vi "BPZ V1.5.vi"() -> ()   [LabVIEW 2025]
uses:
  StatesV2.0.ctl
  runningPhaseV2.0.ctl
  CommandsV2.0.ctl
  <vilib>/Analysis/3filter.llb/Filter Passband Type.ctl
  <vilib>/Utility/error.llb/DialogType.ctl
  <vilib>/Utility/file.llb/Write Delimited Spreadsheet (DBL).vi
  <vilib>/Instr/_visa.llb/VISA Configure Serial Port (Instr).vi
  <vilib>/Analysis/NI_AALBase.lvlib
  <vilib>/ptbypt/NI_PtbyPt.lvlib
panel:
  out "Time working":dbl format="%<%H:%M:%S>t"
  out "State":T1
  out "Current time":timestamp format="%<%H:%M:%S\n%x>T"
  in  "Em. Stop":bool
  out "Drive torque [mNm]":dbl(knob)=4657.939556380271 scale=0.0..1000.0 scale format="%#_2f"
  out "Motor velocity [RPM]":dbl(knob) scale=0.0..800.0
  out "Motor current [A]":dbl(knob) scale=0.0..5.0
  out "Gear temperature":dbl(slide)=24.329999999999984 scale=0.0..200.0
  out "Amb. temperature":dbl(slide)=24.970000000000027 scale=0.0..50.0
  out "Noise level [dB]":dbl(knob)=36.22 scale=0.0..120.0
  out "Automatic on":bool
  out "UART status":bool=TRUE
  out "Pump 1 engaged":bool
  out "Pump 2 engaged":bool
  out "Logging":bool
  out "Drive on":bool
  out "EPOS Status":bool=TRUE
  in  "?":T2(tab)=enum."Settings"
  in  "Connect":bool
  in  "Disconnect":bool
  in  "Connect":bool
  in  "Disconnect":bool
  in  "Pump 1":bool
  in  "Pump 2":bool
  in  "Filename":string
  in  "Ready":bool
  in  "Log folder":path
  in  "AutoStop":bool
  in  "AutoStart":bool
  in  "Enable logging":bool
  in  "Current filter":bool
  in  "Array":cluster{"RPM":u16, "TIME [s]":u32}[](array[cluster])
  out "targetRPM":i32
  out "cyclesCompleted":i32
  out "cyclesToComplete":i32
  out "runningPhase":T3
  out "ETA":u32 format="%<%H:%M:%S>t"
  in  "Communication settings":T4={"Device"="EPOS4", "Protocol stack "="MAXON SERIAL V2", "Interface"="USB", "Port"="USB0", "Baud rate"=1000000, "Timeout [ms]"=500}
  in  "Velocity profile":T5={"Acceleration [rpm/s]"=1060, "Deceleration  [rpm/s]"=1060}
  in  "UART Settings":T6={"Flow control"=0, "Stop bits"=10, "Parity bit"=enum."None", "Data bits"=8, "Baud rate"=115200, "Port"="COM3"} {"Stop bits" items=["1.0"=10, "1.5"=15, "2.0"=20]; "Flow control" items=["None", "XON/XOFF", "RTS/CTS", "XON/XOFF & RTS/CTS", "DTR/DSR", "XON/XOFF & DTR/DSR"]}
  in  "Surface emmisivity":dbl=1.0 min=0.05 max=1.0 step=0.05 format="%#.2g"
  in  "Torque constant [mNm/mA]":dbl=0.0273
  in  "Motor gear ratio":dbl=5.3076
  in  "Belt drive ratio":dbl=1.5
  in  "Motor gear efficiency":dbl=0.9
  in  "Belt drive efficiency":dbl=0.95 min=0.89 max=0.99 step=0.01
  in  "Speed setting [RPM]":dbl=60.0 min=0.0 max=750.0 step=10.0
  in  "Stop motor":bool
  in  "Start motor":bool
  in  "Stop logging":bool
  in  "Start logging":bool
  in  "?":T7(tab)
  out "Velocity [RPM]":cluster{dbl[], dbl[]}(graph)
  out "Torque [mNm]":cluster{dbl[], dbl[]}(graph)
  out "Noise [dB]":cluster{dbl[], dbl[]}(graph)
  out "Temperature [degC]":cluster{dbl[], dbl[]}[](graph)
  in  "QUIT":bool
  # "Current status"
  # "EPOS connection control"
  # "UART connection control"
  # "Pump control"
  # "Options"
  # "Start/Stop"
  # "EPOS Settings"
  # "UART Settings"
  # "Motor control"
  # "Logger control"
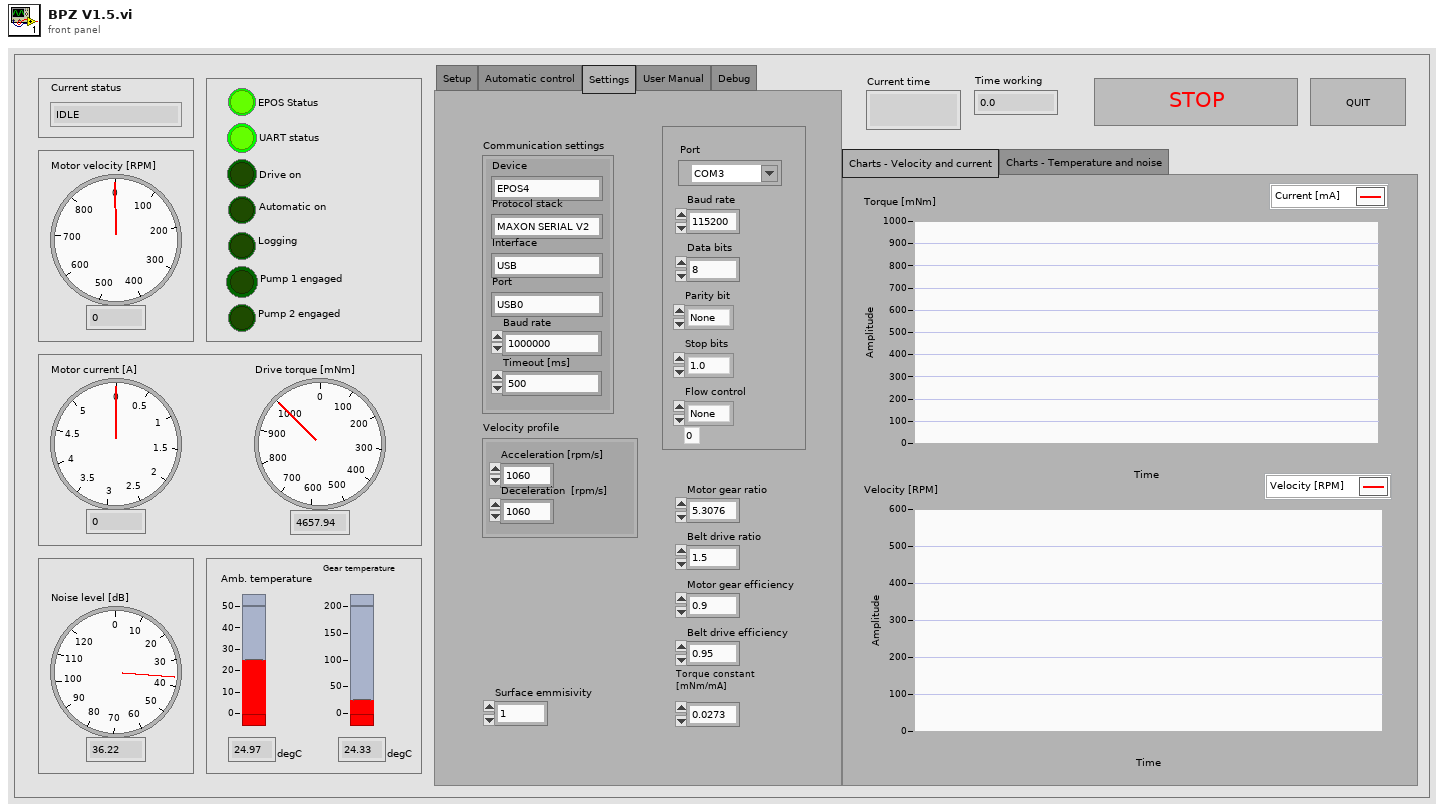
[diagram p1: front panel]
types:
  T1 = typedef "StatesV2.0.ctl" = enum16{"IDLE", "READY", "RUNNING", "ERROR", "SHUTDOWN"}
  T2 = enum32{"Setup", "Automatic control", "Settings", "User Manual", "Debug"}
  T3 = typedef "runningPhaseV2.0.ctl" = enum16{"DISABLED", "INITIALIZE_CYCLE", "START_MOTOR", "COUNTDOWN", "STOP_MOTOR", "CYCLE_COMPLETE"}
  T4 = cluster{"Device":string, "Protocol stack ":string, "Interface":string, "Port":string, "Baud rate":u32, "Timeout [ms]":u32}
  T5 = cluster{"Acceleration [rpm/s]":u32, "Deceleration  [rpm/s]":u32}
  T6 = cluster{"Flow control":u16, "Stop bits":u16, "Parity bit":enum16{"None", "Odd", "Even", "Mark", "Space"}, "Data bits":u16, "Baud rate":u32, "Port":refnum<visa-resource-name>}
  T7 = enum32{"Charts - Velocity and current", "Charts - Temperature and noise"}
  T8 = cluster{"UART":cluster{"Amb. temp":dbl[], "Gear temp":dbl[], "Noise lvl":dbl[], "time":dbl[]}, "EPOS":cluster{"Speed":dbl[], "Torque":dbl[], "time":dbl[]}}
  T9 = typedef "CommandsV2.0.ctl" = enum16{"No_Command", "Ready", "Initialize_Cycle", "Stop", "SHUTDOWN", "EPOS_Connect", "EPOS_Disconnect", "UART_Connect", "UART_Disconnect", "Pump1_Toggle", "Pump2_Toggle"}
  T10 = cluster{"Speed":dbl[], "Torque":dbl[], "time":dbl[]}
  T11 = typedef "NI_AALBase.lvlib/Filter Passband Type.ctl" = enum32{"Lowpass", "Highpass", "Bandpass", "Bandstop"}
  T12 = cluster{"Gear temp":dbl, "Amb temp":dbl, "Noise lvl":dbl, "Torque":dbl, "RPM":dbl, "Time":dbl}
  T13 = cluster{"isLoggingEnabled":bool, "isUARTConnected":bool, "isEPOSConnected ":bool, "lastCommand":T9, "cyclesToComplete":i32, "targetRPM":i32, "axisHandle":cluster{"keyHandle":u32, "nodeId":u16}, "VISA resource name":refnum<visa-resource-name>, "isMotorOn":bool, "runningPhase":T3, "cyclesCompleted":i32, "isPump1on":bool, "isPump2on":bool, "timeToComplete":u32, "lastNotifyMs":u32, "UARTStartTime":timestamp, "MotorStartTime":timestamp, "ETA":u32}
  T14 = cluster{"Amb. temp":dbl[], "Gear temp":dbl[], "Noise lvl":dbl[], "time":dbl[]}
  T15 = cluster{"array type (2D Dbl)[0]":dbl, "array type (2D Dbl)[1]":dbl, "array type (2D Dbl)[2]":dbl}
  T16 = typedef "DialogType.ctl" = u16
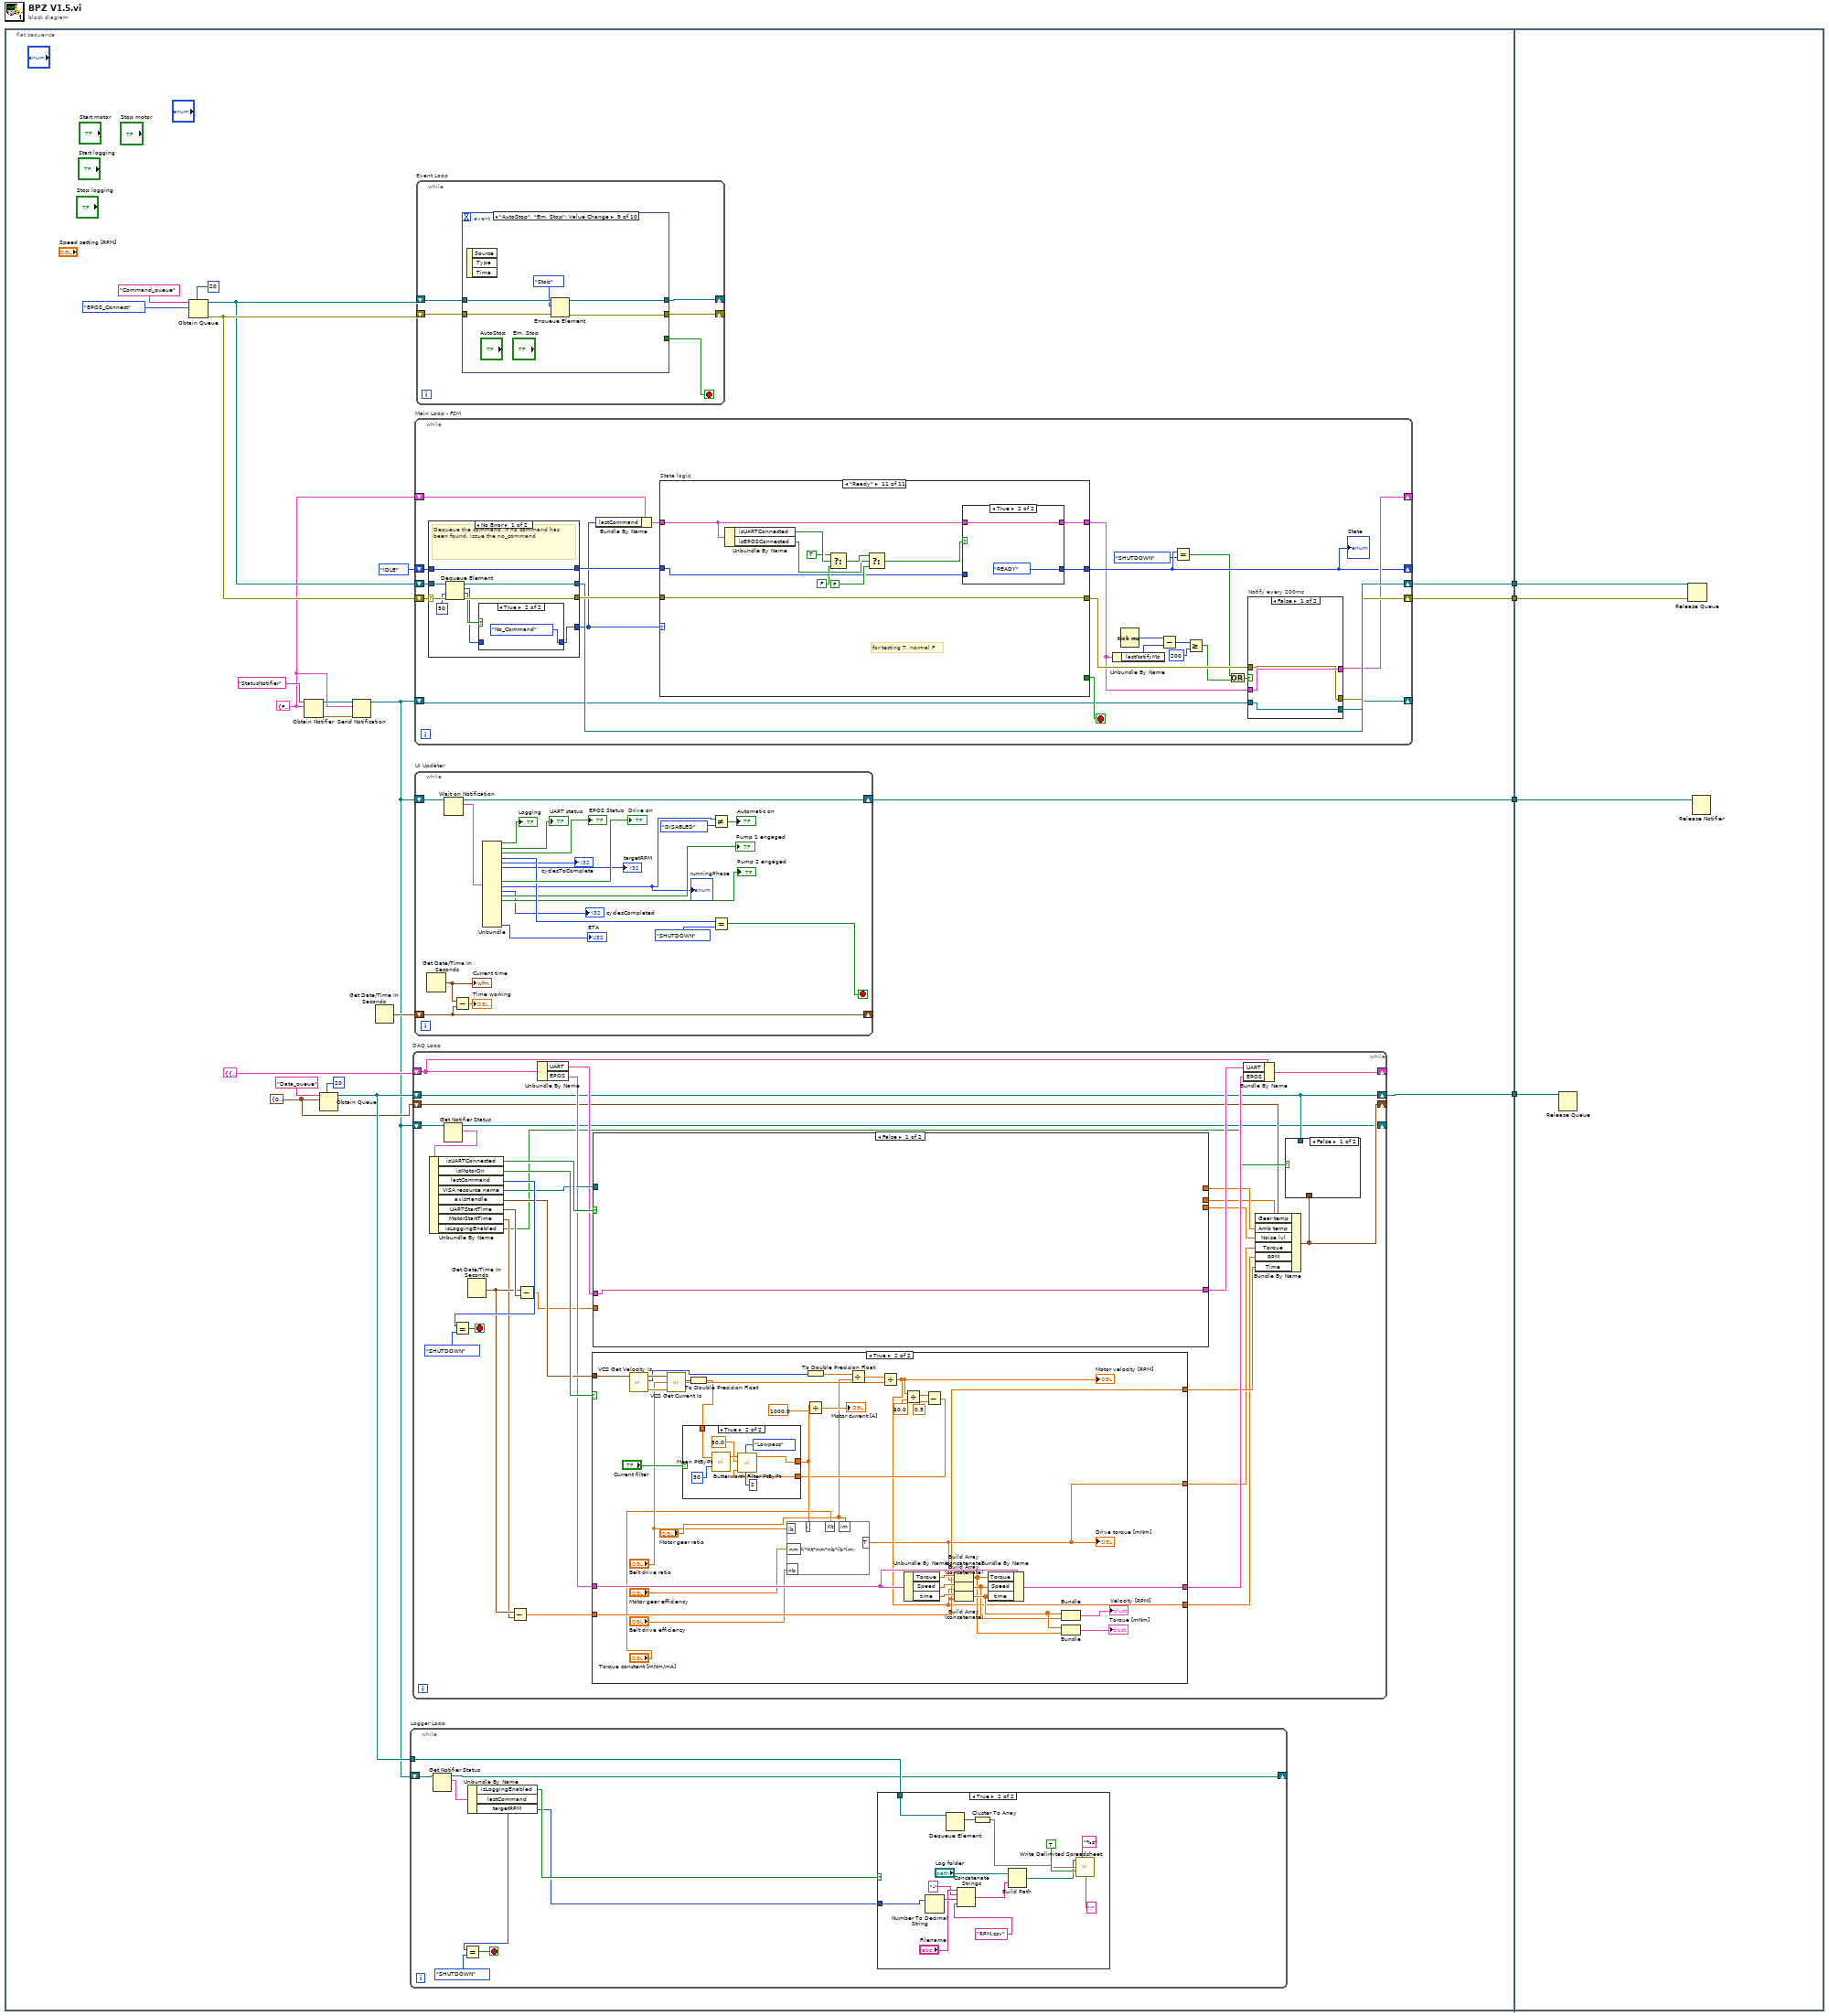
[diagram p0: block diagram]
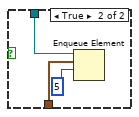
[diagram p3: hidden frame]
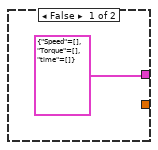
[diagram p4: hidden frame]
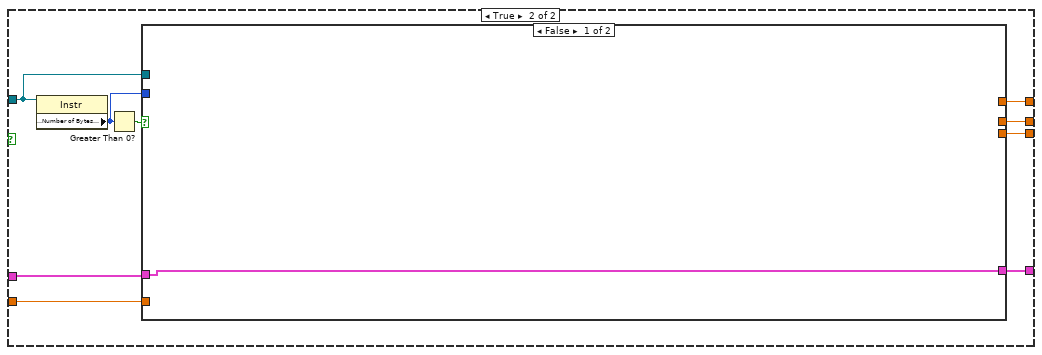
[diagram p6: hidden frame]
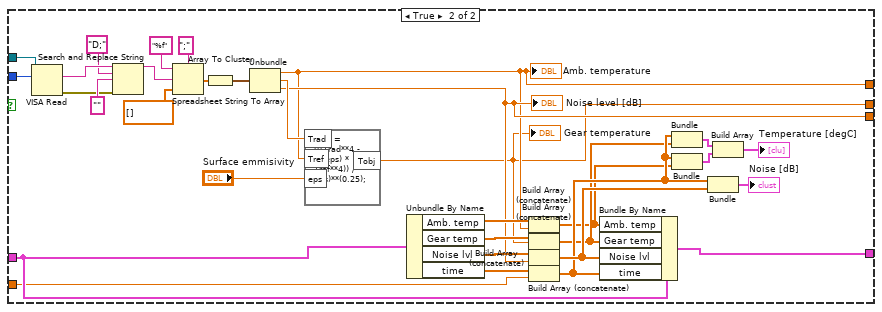
[diagram p7: hidden frame]
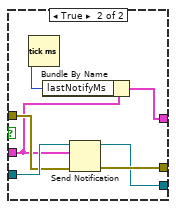
[diagram p8: hidden frame]
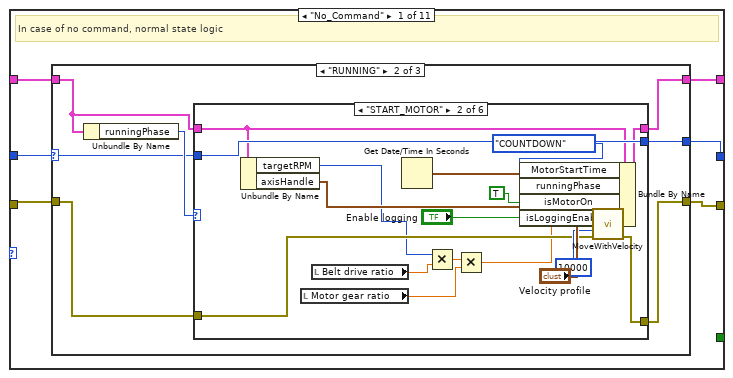
[diagram p9: hidden frame]
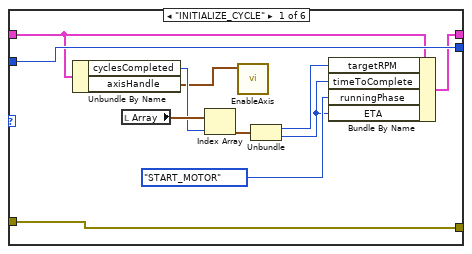
[diagram p11: hidden frame]
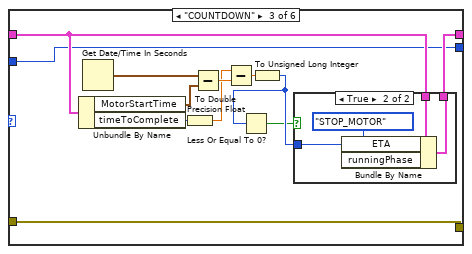
[diagram p12: hidden frame]
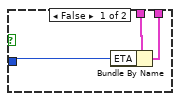
[diagram p13: hidden frame]
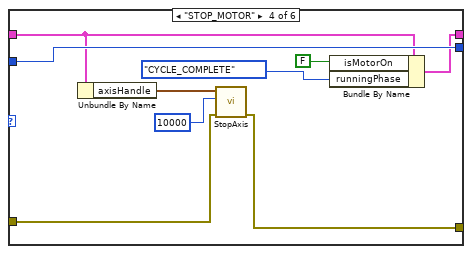
[diagram p14: hidden frame]
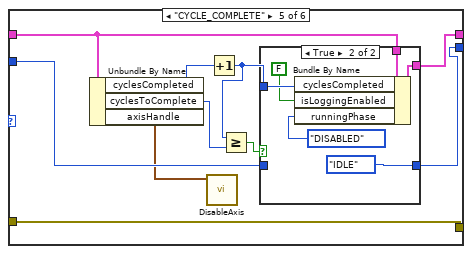
[diagram p15: hidden frame]
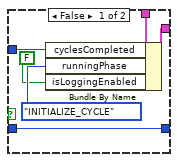
[diagram p16: hidden frame]
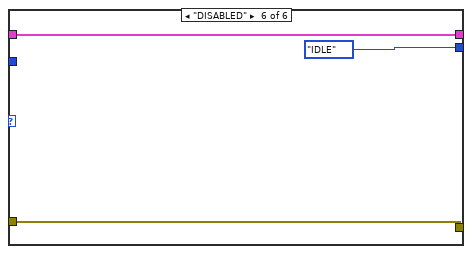
[diagram p17: hidden frame]
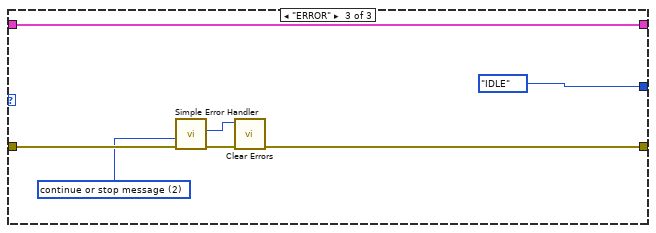
[diagram p18: hidden frame]
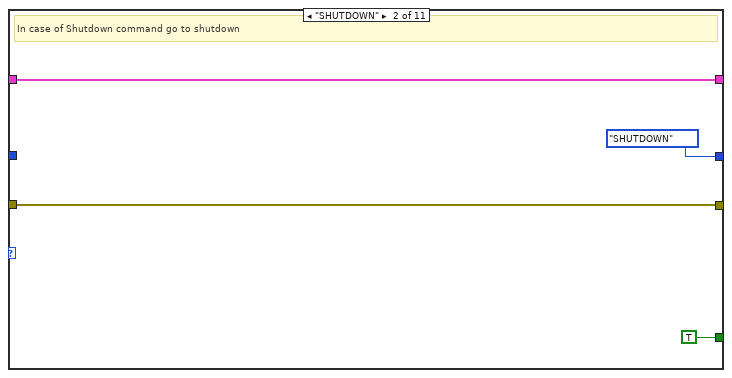
[diagram p19: hidden frame]
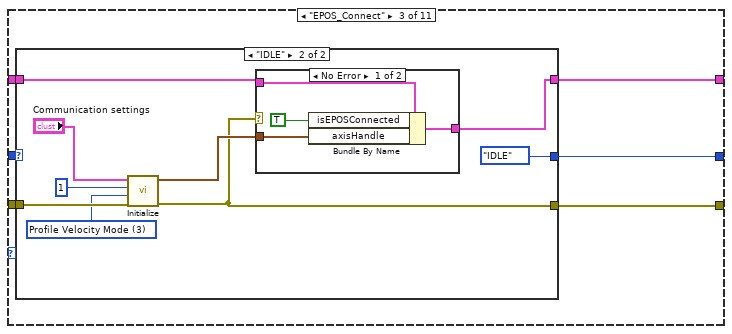
[diagram p20: hidden frame]
diagram:
  n1 = flat-sequence {
    tunnel: [w19] -> w4
    tunnel: [w7] -> w3
    tunnel: [w6] -> w2
    tunnel: [w5] -> w1
    tunnel: w4 -> [w550]
    tunnel: w3 -> [w549]
    tunnel: w2 -> [w548]
    tunnel: w1 -> [w547]
    frame #0 {
      w14 = T12 {"Gear temp"=0.0, "Amb temp"=0.0, "Noise lvl"=0.0, "Torque"=0.0, "RPM"=0.0, "Time"=0.0}
      w8 = T13 {"isLoggingEnabled"=FALSE, "isUARTConnected"=FALSE, "isEPOSConnected "=FALSE, "lastCommand"=enum."No_Command", "cyclesToComplete"=0, "targetRPM"=0, "axisHandle"={"keyHandle"=0, "nodeId"=1}, "VISA resource name"="", "isMotorOn"=FALSE, "runningPhase"=enum."DISABLED", "cyclesCompleted"=0, "isPump1on"=FALSE, "isPump2on"=FALSE, "timeToComplete"=0, "lastNotifyMs"=0, "UARTStartTime"=timestamp(0 s since 1904-01-01), "MotorStartTime"=timestamp(0 s since 1904-01-01), "ETA"=0}
      n2 = Obtain Queue(max queue size (-1, unlimited)=20, name (unnamed)="Command_queue", element data type=CommandsV2.0."EPOS_Connect") -> (queue out=w22:refnum<queue>, error out=w23:errorcluster)  [unwired: 2 in, 1 out]
      n3 = Obtain Notifier(name (unnamed)="StatusNotifier", notification data type=w8) -> (notifier out=w11:refnum<notifier>, error out=w9:errorcluster)  [unwired: 2 in, 1 out]
      n4 = Obtain Queue(max queue size (-1, unlimited)=20, name (unnamed)="Data_queue", element data type=w14) -> (queue out=w15:refnum<queue>)  [unwired: 2 in, 2 out]
      n5 = Send Notification(notification=w8, notifier=w11, error in (no error)=w9) -> (notifier out=w10:refnum<notifier>)  [unwired: 1 out]
      n6 = Get Date/Time In Seconds() -> (seconds since 1Jan1904=w18:timestamp)
      n7 = while "Logger Loop" {
        tunnel: w15 -> [w34]
        shift-right: [w29] -> _
        shift-left: w10 -> [w30]
        stop <- w32 stop-if-true
        n8 = Get Notifier Status(notifier=w30) -> (notifier out=w29:refnum<notifier>, current notification=w28:T13)  [unwired: 1 in, 3 out]
        n9 = Unbundle By Name(w28) -> ("isLoggingEnabled"=w27:bool, "lastCommand"=w31:T9, "targetRPM"=w26:i32)
        n10 = Equal?(x=w31, y=CommandsV2.0."SHUTDOWN") -> (x = y?=w32:bool)
        n11 = case shown="True" w27 {
          tunnel: w34 -> [_ w48]
          tunnel: w26 -> [_ w46]
          frame False {
          }
          frame True {
            n12 = Number To Decimal String(number=w46) -> (decimal integer string=w45:string)  [unwired: 1 in]
            n13 = Dequeue Element(queue=w48) -> (element=w41:T12)  [unwired: 2 in, 3 out]
            n14 = Concatenate Strings("Filename", "-" ("string"), w45, "RPM.csv" ("string")) -> (w43:string)
            n15 = Cluster To Array(cluster=w41) -> (array=w40:dbl[])
            n16 = Build Path(base path="Log folder", name or relative path=w43) -> (appended path=w38:path)
            n17 = call-poly <vilib>:"Write Delimited Spreadsheet.vi"("file path (dialog if empty)"=w38, "format (%.3f)"="%s", "1D data"=w40, "append to file? (new file:F)"=TRUE, "delimiter (\\t)"=";" ("delimiter (\\t)")) -> ()  [unwired: 9 in, 2 out]
          }
        }
      }
      n18 = while "DAQ Loop" {
        shift-right: [w50] -> _
        shift-left: w10 -> [w51]
        shift-right: [w62] -> _
        shift-left: T8 {"UART"={"Amb. temp"=[], "Gear temp"=[], "Noise lvl"=[], "time"=[]}, "EPOS"={"Speed"=[], "Torque"=[], "time"=[]}} -> [w72]
        shift-right: [w60] -> w5
        shift-left: w15 -> [w60]
        shift-right: [w52] -> _
        shift-left: w14 -> [w59]
        stop <- w77 stop-if-true
        n19 = Get Notifier Status(notifier=w51) -> (notifier out=w50:refnum<notifier>, current notification=w49:T13)  [unwired: 1 in, 3 out]
        n20 = Unbundle By Name(w49) -> ("isUARTConnected"=w75:bool, "isMotorOn"=w76:bool, "lastCommand"=w78:T9, "VISA resource name"=w74:refnum<visa-resource-name>, "axisHandle"=w70:cluster{"keyHandle":u32, "nodeId":u16}, "UARTStartTime"=w67:timestamp, "MotorStartTime"=w65:timestamp, "isLoggingEnabled"=w61:bool)
        n21 = Equal?(x=w78, y=CommandsV2.0."SHUTDOWN") -> (x = y?=w77:bool)
        n22 = Get Date/Time In Seconds() -> (seconds since 1Jan1904=w66:timestamp)
        n23 = Subtract(x=w66, y=w65) -> (x-y=w64:dbl)
        n24 = Subtract(x=w66, y=w67) -> (x-y=w68:dbl)
        n25 = Unbundle By Name(w72) -> ("UART"=w73:T14, "EPOS"=w69:T10)
        n26 = case shown="True" w76 {
          tunnel: w70 -> [_ w116]
          tunnel: w69 -> [_ w104]
          tunnel: w64 -> [_ w96]
          tunnel: [T10 {"Speed"=[], "Torque"=[], "time"=[]} ("EPOS") w100] -> w63
          tunnel: [_ w96] -> w58
          tunnel: [_ w95] -> w57
          tunnel: [_ w94] -> w56
          frame False {
          }
          frame True {
            n27 = call "VCS Get Velocity Is.vi"("axis in"=w116) -> ("error out"=w112:errorcluster, "velocityIs"=w110:i32, "axis out"=w117:cluster{"keyHandle":u32, "nodeId":u16})  [unwired: 8 in]
            n28 = call "VCS Get Current Is.vi"("error in (no error)"=w112, "axis in"=w117) -> ("currentIs"=w88:i16)  [unwired: 7 in, 2 out]
            n29 = To Double Precision Float(number=w88) -> (double precision float=w86:dbl)
            n30 = To Double Precision Float(number=w110) -> (double precision float=w87:dbl)
            n31 = Divide(x=w87, y="Motor gear ratio") -> (x/y=w109:dbl)
            n32 = Divide(x=w109, y="Belt drive ratio") -> (x/y=w95:dbl)
            "Motor velocity [RPM]" <- w95
            n33 = Unbundle By Name(w104) -> ("Torque"=w103:dbl[], "Speed"=w102:dbl[], "time"=w101:dbl[])
            n34 = Divide(x=w95, y=60.0) -> (x/y=w107:dbl)
            n35 = Subtract(x=w107, y=0.5) -> (x-y=w105:dbl)
            n36 = case shown="True" "Current filter" {
              tunnel: w105 -> [_ w121]
              tunnel: [w118 w119] -> w111
              tunnel: w86 -> [w118 w120]
              frame False {
              }
              frame True {
                n37 = call <vilib>:"Mean PtByPt.vi"("x"=w120, "sample length"=30) -> ("mean"=w125:dbl)  [unwired: 2 in, 1 out]
                n38 = call <vilib>:"Butterworth Filter PtByPt.vi"("order"=2, "filter type"=Filter_Passband_Type."Lowpass", "low cutoff freq: fl"=w121, "sampling freq: fs"=50.0, "x"=w125) -> ("Filtered x"=w119:dbl)  [unwired: 4 in, 1 out]
              }
            }
            n39 = formula code="T =i*Kt*nm*nb*ib*im;"("nb"="Belt drive efficiency", "nm"="Motor gear efficiency", "ib"="Belt drive ratio", "im"="Motor gear ratio", "i"=w111, "Kt"="Torque constant [mNm/mA]") -> ("T"=w94:dbl)
            "Drive torque [mNm]" <- w94
            n40 = Divide(x=w111, y=1000.0) -> (x/y=→"Motor current [A]":dbl)
            n41 = Build Array (concatenate)(w103, w94) -> (w97:dbl[])
            n42 = Build Array (concatenate)(w102, w95) -> (w98:dbl[])
            n43 = Build Array (concatenate)(w101, w96) -> (w99:dbl[])
            n44 = Bundle By Name(cluster=w104, "Torque"=w97, "Speed"=w98, "time"=w99) -> (w100:T10)
            n45 = Bundle(w99, w98) -> (→"Velocity [RPM]":cluster{dbl[], dbl[]})  [unwired: 1 in]
            n46 = Bundle(w99, w97) -> (→"Torque [mNm]":cluster{dbl[], dbl[]})  [unwired: 1 in]
          }
        }
        n47 = case shown="False" w75 {
          tunnel: w74 -> [_ w135]
          tunnel: w73 -> [w127 w134]
          tunnel: [w127 w133] -> w71
          tunnel: w68 -> [_ w131]
          tunnel: [_ w130] -> w55
          tunnel: [_ w129] -> w54
          tunnel: [_ w128] -> w53
          frame False {
          }
          frame True {
            n48 = property class="Instr"(reference=w135) -> ("Serial Settings:Number of Bytes at Serial Port"=w132:u32)  [unwired: 1 in, 2 out]
            n49 = Greater Than 0?(x=w132) -> (x > 0?=w136:bool)
            n50 = case shown="False" w136 {
              tunnel: w135 -> [_ w169]
              tunnel: w134 -> [w137 w153]
              tunnel: [w137 w151] -> w133
              tunnel: w132 -> [_ w150]
              tunnel: w131 -> [_ w141]
              tunnel: [_ w140] -> w130
              tunnel: [_ w139] -> w129
              tunnel: [_ w138] -> w128
              frame False {
              }
              frame True {
                n51 = VISA Read(VISA resource name=w169, byte count=w150) -> (read buffer=w168:string, error out=w165:errorcluster)  [unwired: 1 in, 2 out]
                n52 = Search and Replace String(input string=w168, search string="D;", replace string="" ("replace string (\"\")"), error in=w165) -> (result string=w164:string)  [unwired: 4 in, 3 out]
                n53 = Spreadsheet String To Array(delimiter (Tab)=";", format string="%f", spreadsheet string=w164, array type (2D Dbl)=dbl[] []) -> (array=w161:dbl[])
                n54 = Array To Cluster(array=w161) -> (cluster=w159:T15)
                n55 = Unbundle(w159) -> ("array type (2D Dbl)[0]"=w139:dbl, "array type (2D Dbl)[1]"=w158:dbl, "array type (2D Dbl)[2]"=w140:dbl)
                "Noise level [dB]" <- w140
                "Amb. temperature" <- w139
                n56 = formula code="Tobj = (((Trad**4 - (1-eps) * Tref**4)) / eps)**(0.25);"("Trad"=w158, "Tref"=w139, "eps"="Surface emmisivity") -> ("Tobj"=w138:dbl)
                "Gear temperature" <- w138
                n57 = Unbundle By Name(w153) -> ("Amb. temp"=w156:dbl[], "Gear temp"=w155:dbl[], "Noise lvl"=w154:dbl[], "time"=w152:dbl[])
                n58 = Build Array (concatenate)(w156, w139) -> (w145:dbl[])
                n59 = Build Array (concatenate)(w155, w138) -> (w146:dbl[])
                n60 = Build Array (concatenate)(w154, w140) -> (w149:dbl[])
                n61 = Build Array (concatenate)(w152, w141) -> (w147:dbl[])
                n62 = Bundle By Name(cluster=w153, "Amb. temp"=w145, "Gear temp"=w146, "Noise lvl"=w149, "time"=w147) -> (w151:T14)
                n63 = Bundle(w147, w146) -> (w143:cluster{dbl[], dbl[]})  [unwired: 1 in]
                n64 = Bundle(w147, w145) -> (w144:cluster{dbl[], dbl[]})  [unwired: 1 in]
                n65 = Bundle(w147, w149) -> (→"Noise [dB]":cluster{dbl[], dbl[]})  [unwired: 1 in]
                n66 = Build Array(w143, w144) -> (→"Temperature [degC]":cluster{dbl[], dbl[]}[])
              }
            }
          }
        }
        n67 = Bundle By Name(cluster=w72, "UART"=w71, "EPOS"=w63) -> (w62:T8)
        n68 = Bundle By Name(cluster=w59, "Gear temp"=w53, "Amb temp"=w54, "Noise lvl"=w55, "Torque"=w56, "RPM"=w57, "Time"=w58) -> (w52:T12)
        n69 = case shown="False" w61 {
          tunnel: w60 -> [_ w82]
          tunnel: w52 -> [_ w81]
          frame False {
          }
          frame True {
            n70 = Enqueue Element(queue=w82, element=w81, timeout in ms (-1)=5) -> ()  [unwired: 1 in, 3 out]
          }
        }
      }
      n71 = while "Main Loop - FSM" {
        shift-right: [w206] -> w6
        shift-left: w23 -> [w216]
        shift-right: [w210] -> w7
        shift-left: w22 -> [w215]
        shift-right: [w201] -> _
        shift-left: StatesV2.0."IDLE" ("currentState") -> [w212]
        shift-right: [w208] -> _
        shift-left: w10 -> [w209]
        shift-right: [w202] -> _
        shift-left: w8 -> [w204]
        stop <- w214 stop-if-true
        n72 = case shown="No Error" w216 {
          selector: w216 -> [w483 w490]
          tunnel: w215 -> [w484 w488]
          tunnel: [w482 w490] -> w213
          tunnel: w212 -> [w478 _]
          tunnel: [w478 StatesV2.0."ERROR" ("currentState")] -> w211
          tunnel: [w477 CommandsV2.0."No_Command"] -> w205
          tunnel: [w476 w488] -> w210
          frame No Error {
            # "Dequeue the command. If no command has been found, issue the no_command"
            n73 = Dequeue Element(queue=w484, timeout in ms (-1)=50, error in (no error)=w483) -> (queue out=w476:refnum<queue>, element=w480:T9, timed out?=w481:bool, error out=w482:errorcluster)
            n74 = case shown="True" w481 {
              tunnel: w480 -> [w485 _]
              tunnel: [w485 CommandsV2.0."No_Command"] -> w477
              frame False {
              }
              frame True {
              }
            }
          }
          frame Error {
          }
        }
        n75 = Bundle By Name(cluster=w204, "lastCommand"=w205) -> (w203:T13)
        n76 = case "State logic" shown="\"Ready\"" w205 {
          tunnel: [w229 StatesV2.0."SHUTDOWN" ("currentState") w338 StatesV2.0."IDLE" ("currentState") w371 StatesV2.0."IDLE" ("currentState") w405 w426 w455 w457 w470] -> w201
          tunnel: w211 -> [w232 _ w335 _ w369 _ w410 w427 w455 w457 w459]
          tunnel: [_ TRUE _ _ _ _ _ _ _ _ _] -> w214
          tunnel: w203 -> [w231 w331 w337 w361 w372 w401 w409 w425 w453 w456 w466]
          tunnel: [w230 w331 w336 w359 w373 w399 w408 w424 w453 w456 w469] -> w197
          tunnel: w213 -> [w228 w332 w340 w363 w370 w404 w407 w423 w454 w458 w468]
          tunnel: [w227 w332 w339 w364 w368 w403 w406 w422 w454 w458 w468] -> w207
          frame "No_Command" {
            # "In case of no command, normal state logic"
            n77 = case shown="\"RUNNING\"" w232 {
              selector: w232 -> [w234 w241 _]
              tunnel: w231 -> [w235 w237 w330]
              tunnel: [w235 w236 w330] -> w230
              tunnel: [w234 w240 StatesV2.0."IDLE" ("currentState")] -> w229
              tunnel: w228 -> [w233 w239 w327]
              tunnel: [w233 w238 w326] -> w227
              frame Default {
              }
              frame "RUNNING" {
                n78 = Unbundle By Name(w237) -> ("runningPhase"=w242:T3)
                n79 = case shown="\"START_MOTOR\"" w242 {
                  tunnel: w241 -> [w252 w270 w272 w298 w303 _]
                  tunnel: [w252 w270 w272 w298 w304 StatesV2.0."IDLE" ("currentState")] -> w240
                  tunnel: w239 -> [w253 w261 w282 w296 w308 w321]
                  tunnel: [w253 w267 w282 w295 w308 w321] -> w238
                  tunnel: w237 -> [w250 w266 w276 w294 w302 w322]
                  tunnel: [w247 w264 w275 w293 w301 w322] -> w236
                  frame "INITIALIZE_CYCLE" {
                    n80 = Unbundle By Name(w250) -> ("cyclesCompleted"=w245:i32, "axisHandle"=w243:cluster{"keyHandle":u32, "nodeId":u16})
                    n81 = local read "Array"() -> (w251:cluster{"RPM":u16, "TIME [s]":u32}[])
                    n82 = Index Array(array=w251, index=w245) -> (element=w249:cluster{"RPM":u16, "TIME [s]":u32})
                    n83 = call "EnableAxis.vi"("axis in"=w243) -> ()  [unwired: 5 in, 2 out]
                    n84 = Unbundle(w249) -> ("RPM"=w248:u16, "TIME [s]"=w244:u32)
                    n85 = Bundle By Name(cluster=w250, "targetRPM"=w248, "timeToComplete"=w244, "runningPhase"=runningPhaseV2.0."START_MOTOR", "ETA"=w244) -> (w247:T13)
                  }
                  frame "START_MOTOR" {
                    n86 = Unbundle By Name(w266) -> ("targetRPM"=w259:i32, "axisHandle"=w262:cluster{"keyHandle":u32, "nodeId":u16})
                    n87 = local read "Motor gear ratio"() -> (w255:dbl)
                    n88 = local read "Belt drive ratio"() -> (w256:dbl)
                    n89 = Get Date/Time In Seconds() -> (seconds since 1Jan1904=w265:timestamp)
                    n90 = Multiply(x=w259, y=w256) -> (x*y=w260:dbl)
                    n91 = Multiply(x=w260, y=w255) -> (x*y=w258:dbl)
                    n92 = Bundle By Name(cluster=w266, "MotorStartTime"=w265, "runningPhase"=runningPhaseV2.0."COUNTDOWN", "isMotorOn"=TRUE, "isLoggingEnabled"="Enable logging") -> (w264:T13)
                    n93 = call "MoveWithVelocity.vi"("axis in"=w262, "velocity profile"="Velocity profile", "targetVelocity"=w258, "timeout"=u32 10000, "error in (no error)"=w261) -> ("error out"=w267:errorcluster)  [unwired: 9 in, 1 out]
                  }
                  frame "COUNTDOWN" {
                    n94 = Unbundle By Name(w276) -> ("MotorStartTime"=w281:timestamp, "timeToComplete"=w278:u32)
                    n95 = Get Date/Time In Seconds() -> (seconds since 1Jan1904=w280:timestamp)
                    n96 = To Double Precision Float(number=w278) -> (double precision float=w277:dbl)
                    n97 = Subtract(x=w280, y=w281) -> (x-y=w279:dbl)
                    n98 = Subtract(x=w277, y=w279) -> (x-y=w274:dbl)
                    n99 = To Unsigned Long Integer(number=w274) -> (unsigned 32bit integer=w273:u32)
                    n100 = Less Or Equal To 0?(x=w273) -> (x <= 0?=w271:bool)
                    n101 = case shown="True" w271 {
                      tunnel: w276 -> [w285 w289]
                      tunnel: [w284 w288] -> w275
                      tunnel: w273 -> [w283 w287]
                      frame False {
                        n102 = Bundle By Name(cluster=w285, "ETA"=w283) -> (w284:T13)
                      }
                      frame True {
                        n103 = Bundle By Name(cluster=w289, "ETA"=w287, "runningPhase"=runningPhaseV2.0."STOP_MOTOR") -> (w288:T13)
                      }
                    }
                  }
                  frame "STOP_MOTOR" {
                    n104 = Unbundle By Name(w294) -> ("axisHandle"=w297:cluster{"keyHandle":u32, "nodeId":u16})
                    n105 = call "StopAxis.vi"("error in (no error)"=w296, "timeout"=u32 10000, "axis in"=w297) -> ("error out"=w295:errorcluster)  [unwired: 3 in, 1 out]
                    n106 = Bundle By Name(cluster=w294, "isMotorOn"=FALSE, "runningPhase"=runningPhaseV2.0."CYCLE_COMPLETE") -> (w293:T13)
                  }
                  frame "CYCLE_COMPLETE" {
                    n107 = Unbundle By Name(w302) -> ("cyclesCompleted"=w307:i32, "cyclesToComplete"=w306:i32, "axisHandle"=w299:cluster{"keyHandle":u32, "nodeId":u16})
                    n108 = call "DisableAxis.vi"("axis in"=w299) -> ()  [unwired: 5 in, 2 out]
                    n109 = Increment(x=w307) -> (x+1=w300:i32)
                    n110 = Greater Or Equal?(x=w300, y=w306) -> (x >= y?=w305:bool)
                    n111 = case shown="True" w305 {
                      tunnel: [w314 StatesV2.0."IDLE" ("currentState")] -> w304
                      tunnel: w303 -> [w314 _]
                      tunnel: w302 -> [w313 w318]
                      tunnel: w300 -> [w312 w319]
                      tunnel: [w311 w317] -> w301
                      frame False {
                        n112 = Bundle By Name(cluster=w313, "cyclesCompleted"=w312, "runningPhase"=runningPhaseV2.0."INITIALIZE_CYCLE", "isLoggingEnabled"=FALSE) -> (w311:T13)
                      }
                      frame True {
                        n113 = Bundle By Name(cluster=w318, "cyclesCompleted"=w319, "isLoggingEnabled"=FALSE ("isPump1on"), "runningPhase"=runningPhaseV2.0."DISABLED") -> (w317:T13)
                      }
                    }
                  }
                  frame "DISABLED" {
                  }
                }
              }
              frame "ERROR" {
                w325 = T16 2 items=["no dialog", "OK message", "continue or stop message", "OK message + warnings", "continue/stop + warnings"] ("type of dialog (OK msg:1)")
                n114 = call <vilib>:"Simple Error Handler.vi"("type of dialog (OK msg:1)"=w325, "error in (no error)"=w327) -> ("code out"=w328:i32, "error out"=w329:errorcluster)  [unwired: 3 in, 3 out]
                n115 = call <vilib>:"Clear Errors.vi"("error in (no error)"=w329, "specific error code to clear (0: all)"=w328) -> ("error out"=w326:errorcluster)  [unwired: 4 in, 1 out]
              }
            }
          }
          frame "SHUTDOWN" {
            # "In case of Shutdown command go to shutdown"
          }
          frame "EPOS_Connect" {
            n116 = case shown="\"IDLE\"" w335 {
              selector: w335 -> [w342 _]
              tunnel: w340 -> [w341 w352]
              tunnel: [w341 w344] -> w339
              tunnel: [w342 StatesV2.0."IDLE" ("currentState")] -> w338
              tunnel: w337 -> [w343 w351]
              tunnel: [w343 w347] -> w336
              frame Default {
              }
              frame "IDLE" {
                w349 = i8 3 items=["Profile Position Mode"=1, "Profile Velocity Mode"=3, "Homing Mode"=6, "Interpolated Position Mode"=7, "Position Mode"=-1, "Velocity Mode"=-2, "Current Mode"=-3, "Master Encoder Mode"=-5, "Step Direction Mode"=-6] ("modes of operations")
                n117 = call "Initialize.vi"("error in (no error)"=w352, "modes of operations"=w349, "nodeId"=u16 1, "communication settings in"="Communication settings") -> ("error out"=w344:errorcluster, "axis out"=w345:cluster{"keyHandle":u32, "nodeId":u16})  [unwired: 6 in]
                n118 = case shown="No Error" w344 {
                  tunnel: w351 -> [w356 w357]
                  tunnel: w345 -> [w354 _]
                  tunnel: [w353 w357] -> w347
                  frame No Error {
                    n119 = Bundle By Name(cluster=w356, "isEPOSConnected"=TRUE, "axisHandle"=w354) -> (w353:T13)
                  }
                  frame Error {
                  }
                }
              }
            }
          }
          frame "EPOS_Disconnect" {
            n120 = Unbundle By Name(w361) -> ("axisHandle"=w362:cluster{"keyHandle":u32, "nodeId":u16})
            n121 = call "QuickstopAxis.vi"("error in (no error)"=w363, "axis in"=w362) -> ("error out"=w366:errorcluster, "axis out"=w367:cluster{"keyHandle":u32, "nodeId":u16})  [unwired: 4 in]
            n122 = call "DisableAxis.vi"("error in (no error)"=w366, "axis in"=w367) -> ("error out"=w365:errorcluster)  [unwired: 4 in, 1 out]
            n123 = call "Close.vi"("error in (no error)"=w365) -> ("error out"=w364:errorcluster)  [unwired: 10 in]
            n124 = Bundle By Name(cluster=w361, "isEPOSConnected"=FALSE) -> (w359:T13)
          }
          frame "UART_Connect" {
            n125 = case shown="\"IDLE\"" w369 {
              selector: w369 -> [w375 _]
              tunnel: [w376 w381] -> w373
              tunnel: w372 -> [w376 w384]
              tunnel: [w375 StatesV2.0."IDLE" ("currentState")] -> w371
              tunnel: w370 -> [w374 w383]
              tunnel: [w374 w377] -> w368
              frame Default {
              }
              frame "IDLE" {
                n126 = Unbundle("UART Settings") -> ("Flow control"=w390:u16, "Stop bits"=w389:u16, "Parity bit"=w388:enum16{"None", "Odd", "Even", "Mark", "Space"}, "Data bits"=w387:u16, "Baud rate"=w386:u32, "Port"=w385:refnum<visa-resource-name>)
                n127 = call-poly "VISA Configure Serial Port"("VISA resource name"=w385, "baud rate (9600)"=w386, "data bits (8)"=w387, "parity (0:none)"=w388, "error in (no error)"=w383, "stop bits (10: 1 bit)"=w389, "flow control (0:none)"=w390) -> ("VISA resource name out"=w380:refnum<visa-resource-name>, "error out"=w378:errorcluster)  [unwired: 7 in]
                n128 = VISA Flush I/O Buffer(VISA resource name=w380, error in (no error)=w378) -> (VISA resource name out=w379:refnum<visa-resource-name>, error out=w377:errorcluster)  [unwired: 1 in]
                n129 = case shown="No Error" w377 {
                  tunnel: w384 -> [w396 w397]
                  tunnel: w379 -> [w395 _]
                  tunnel: [w394 w397] -> w381
                  frame No Error {
                    n130 = Get Date/Time In Seconds() -> (seconds since 1Jan1904=w392:timestamp)
                    n131 = Bundle By Name(cluster=w396, "VISA resource name"=w395, "isUARTConnected"=TRUE, "UARTStartTime"=w392) -> (w394:T13)
                  }
                  frame Error {
                  }
                }
              }
            }
          }
          frame "UART_Disconnect" {
            n132 = Unbundle By Name(w401) -> ("VISA resource name"=w402:refnum<visa-resource-name>)
            n133 = VISA Close(VISA resource name=w402, error in (no error)=w404) -> (error out=w403:errorcluster)
            n134 = Bundle By Name(cluster=w401, "isUARTConnected"=FALSE) -> (w399:T13)
          }
          frame "Initialize_Cycle" {
            n135 = case shown="\"READY\"" w410 {
              selector: w410 -> [w412 _]
              tunnel: w409 -> [w413 w421]
              tunnel: [w413 w420] -> w408
              tunnel: w407 -> [w411 w416]
              tunnel: [w411 w416] -> w406
              tunnel: [w412 StatesV2.0."RUNNING" ("currentState")] -> w405
              frame Default {
              }
              frame "READY" {
                n136 = Array Size(array="Array") -> (size(s)=w419:i32)
                n137 = Bundle By Name(cluster=w421, "cyclesToComplete"=w419, "cyclesCompleted"=0 ("cycleCount"), "runningPhase"=runningPhaseV2.0."INITIALIZE_CYCLE") -> (w420:T13)
              }
            }
          }
          frame "Stop" {
            n138 = case shown="Default" w427 {
              tunnel: [StatesV2.0."IDLE" ("currentState") StatesV2.0."IDLE" ("currentState")] -> w426
              tunnel: w425 -> [w433 w451]
              tunnel: [w433 w448] -> w424
              tunnel: w423 -> [w430 w449]
              tunnel: [w429 w443] -> w422
              frame Default {
                n139 = Unbundle By Name(w433) -> ("isEPOSConnected"=w432:bool, "axisHandle"=w431:cluster{"keyHandle":u32, "nodeId":u16})
                n140 = case shown="True" w432 {
                  tunnel: w431 -> [_ w441]
                  tunnel: w430 -> [w434 w438]
                  tunnel: [w434 w435] -> w429
                  frame False {
                  }
                  frame True {
                    n141 = call "EnableAxis.vi"("error in (no error)"=w438, "axis in"=w441) -> ("error out"=w439:errorcluster, "axis out"=w440:cluster{"keyHandle":u32, "nodeId":u16})  [unwired: 4 in]
                    n142 = call "StopAxis.vi"("error in (no error)"=w439, "timeout"=u32 5000, "axis in"=w440) -> ("error out"=w436:errorcluster, "axis out"=w437:cluster{"keyHandle":u32, "nodeId":u16})  [unwired: 3 in]
                    n143 = call "DisableAxis.vi"("error in (no error)"=w436, "axis in"=w437) -> ("error out"=w435:errorcluster)  [unwired: 4 in, 1 out]
                  }
                }
              }
              frame "RUNNING" {
                w446 = FALSE ("isLoggingEnabled")
                n144 = Unbundle By Name(w451) -> ("axisHandle"=w450:cluster{"keyHandle":u32, "nodeId":u16})
                n145 = call "StopAxis.vi"("error in (no error)"=w449, "axis in"=w450) -> ("error out"=w444:errorcluster, "axis out"=w445:cluster{"keyHandle":u32, "nodeId":u16})  [unwired: 4 in]
                n146 = call "DisableAxis.vi"("error in (no error)"=w444, "axis in"=w445) -> ("error out"=w443:errorcluster)  [unwired: 4 in, 1 out]
                n147 = Bundle By Name(cluster=w451, "runningPhase"=runningPhaseV2.0."DISABLED", "isLoggingEnabled"=w446, "isMotorOn"=w446) -> (w448:T13)
              }
            }
          }
          frame "Pump1_Toggle" {
          }
          frame "Pump2_Toggle" {
          }
          frame "Ready" {
            # "for testing T, normal F"
            n148 = Unbundle By Name(w466) -> ("isUARTConnected"=w465:bool, "isEPOSConnected"=w464:bool)
            n149 = Select(t=TRUE, s=w465, f=FALSE) -> (s? t:f=w467:bool)
            n150 = Select(t=w467, s=w464, f=FALSE) -> (s? t:f=w460:bool)
            n151 = case shown="True" w460 {
              tunnel: [w473 StatesV2.0."READY" ("currentState")] -> w470
              tunnel: [w472 w474] -> w469
              tunnel: w466 -> [w472 w474]
              tunnel: w459 -> [w473 _]
              frame False {
                n152 = One Button Dialog(message="UART and EPOS need to be connected\n") -> ()  [unwired: 1 in, 1 out]
              }
              frame True {
              }
            }
          }
        }
        "State" <- w201
        n153 = Unbundle By Name(w197) -> ("lastNotifyMs"=w193:u32)
        n154 = Tick Count (ms)() -> (millisecond timer value=w196:u32)
        n155 = Subtract(x=w196, y=w193) -> (x-y=w192:u32)
        n156 = Equal?(x=w201, y=StatesV2.0."SHUTDOWN") -> (x = y?=w199:bool)
        n157 = Greater Or Equal?(x=w192, y=u32 200) -> (x >= y?=w194:bool)
        n158 = Or(x=w199, y=w194) -> (x .or. y?=w198:bool)
        n159 = case "Notify every 200ms" shown="False" w198 {
          tunnel: [w218 w220] -> w202
          tunnel: [w217 w226] -> w206
          tunnel: w197 -> [w218 w222]
          tunnel: w209 -> [w219 w225]
          tunnel: [w219 w224] -> w208
          tunnel: w207 -> [w217 w223]
          frame False {
          }
          frame True {
            n160 = Tick Count (ms)() -> (millisecond timer value=w221:u32)
            n161 = Bundle By Name(cluster=w222, "lastNotifyMs"=w221) -> (w220:T13)
            n162 = Send Notification(notification=w222, notifier=w225, error in (no error)=w223) -> (notifier out=w224:refnum<notifier>, error out=w226:errorcluster)
          }
        }
      }
      n163 = while "UI Updater" {
        shift-right: [w190] -> w19
        shift-left: w10 -> [w191]
        shift-right: [w178] -> _
        shift-left: w18 -> [w178]
        stop <- w181 stop-if-true
        n164 = Get Date/Time In Seconds() -> (seconds since 1Jan1904=w179:timestamp)
        "Current time" <- w179
        n165 = Wait on Notification(notifier=w191) -> (notifier out=w190:refnum<notifier>, notification=w189:T13)  [unwired: 3 in, 2 out]
        n166 = Subtract(x=w179, y=w178) -> (x-y=→"Time working":dbl)
        n167 = Unbundle(w189) -> ("isLoggingEnabled"=→"Logging":bool, "isUARTConnected"=→"UART status":bool, "isEPOSConnected"=→"EPOS Status":bool, "lastCommand"=w180:T9, "cyclesToComplete"=→"cyclesToComplete":i32, "targetRPM"=→"targetRPM":i32, "isMotorOn"=→"Drive on":bool, "runningPhase"=w172:T3, "cyclesCompleted"=→"cyclesCompleted":i32, "isPump1on"=→"Pump 1 engaged":bool, "isPump2on"=→"Pump 2 engaged":bool, "ETA"=→"ETA":u32)  [unwired: 6 out]
        "runningPhase" <- w172
        n168 = Not Equal?(x=w172, y=runningPhaseV2.0."DISABLED") -> (x != y?=→"Automatic on":bool)
        n169 = Equal?(x=w180, y=CommandsV2.0."SHUTDOWN") -> (x = y?=w181:bool)
      }
      n170 = while "Event Loop" {
        shift-right: [w491] -> _
        shift-left: w23 -> [w494]
        shift-right: [w492] -> _
        shift-left: w22 -> [w493]
        stop <- w495 stop-if-true
        n171 = event shown="[8] \"AutoStop\", \"Em. Stop\": Value Change" {
          selector: _ -> [_ _ _ _ _ _ _ _ _ _]
          dyn-events: _ -> [_ _ _ _ _ _ _ _ _ _]
          timeout: _ -> [_ _ _ _ _ _ _ _ _ _]
          tunnel: [_ _ _ _ _ TRUE _ _ _ _] -> w495
          tunnel: [w499 w502 w506 w514 w520 w522 w529 w534 w539 w545] -> w491
          tunnel: w494 -> [w498 w503 w507 w513 w519 w523 w530 w535 w540 w543]
          tunnel: [w500 w504 w509 w515 w518 w525 w528 w533 w538 w546] -> w492
          tunnel: w493 -> [w497 w505 w508 w512 w517 w524 w531 w536 w541 w544]
          event "Connect": Value Change {
            # "EPOS Connect Button"
            n172 = event-data() -> ()  [unwired: 1 in, 2 out]
            n173 = Enqueue Element(queue=w497, element=CommandsV2.0."EPOS_Connect", error in (no error)=w498) -> (queue out=w500:refnum<queue>, error out=w499:errorcluster)  [unwired: 1 in, 1 out]
          }
          event "Pump 1": Value Change {
            n174 = event-data() -> ()  [unwired: 1 in, 2 out]
            n175 = Enqueue Element(queue=w505, element=CommandsV2.0."Pump1_Toggle", error in (no error)=w503) -> (queue out=w504:refnum<queue>, error out=w502:errorcluster)  [unwired: 1 in, 1 out]
          }
          event "Pump 2": Value Change {
            n176 = event-data() -> ()  [unwired: 1 in, 3 out]
            n177 = Enqueue Element(queue=w508, element=CommandsV2.0."Pump2_Toggle", error in (no error)=w507) -> (queue out=w509:refnum<queue>, error out=w506:errorcluster)  [unwired: 1 in, 1 out]
          }
          event "Disconnect": Value Change {
            # "EPOS Disconnect Button"
            n178 = event-data() -> ()  [unwired: 1 in, 2 out]
            n179 = Enqueue Element(queue=w512, element=CommandsV2.0."EPOS_Disconnect", error in (no error)=w513) -> (queue out=w515:refnum<queue>, error out=w514:errorcluster)  [unwired: 1 in, 1 out]
          }
          event "Connect": Value Change {
            # "UART Connect Button"
            n180 = event-data() -> ()  [unwired: 1 in, 2 out]
            n181 = Enqueue Element(queue=w517, element=CommandsV2.0."UART_Connect", error in (no error)=w519) -> (queue out=w518:refnum<queue>, error out=w520:errorcluster)  [unwired: 1 in, 1 out]
          }
          event "QUIT": Value Change {
            n182 = event-data() -> ()  [unwired: 1 in, 3 out]
            n183 = Enqueue Element At Opposite End(queue=w524, element=CommandsV2.0."SHUTDOWN", error in (no error)=w523) -> (queue out=w525:refnum<queue>, error out=w522:errorcluster)  [unwired: 1 in, 1 out]
          }
          event "Ready": Value Change {
            n184 = event-data() -> ()  [unwired: 1 in, 6 out]
            n185 = Enqueue Element(queue=w531, element=CommandsV2.0."Ready", error in (no error)=w530) -> (queue out=w528:refnum<queue>, error out=w529:errorcluster)  [unwired: 1 in, 1 out]
          }
          event "AutoStart": Value Change {
            n186 = event-data() -> ()  [unwired: 1 in, 3 out]
            n187 = Enqueue Element(queue=w536, element=CommandsV2.0."Initialize_Cycle", error in (no error)=w535) -> (queue out=w533:refnum<queue>, error out=w534:errorcluster)  [unwired: 1 in, 1 out]
          }
          event "AutoStop", "Em. Stop": Value Change {
            n188 = event-data() -> ()  [unwired: 1 in, 3 out]
            n189 = Enqueue Element(queue=w541, element=CommandsV2.0."Stop", error in (no error)=w540) -> (queue out=w538:refnum<queue>, error out=w539:errorcluster)  [unwired: 1 in, 1 out]
          }
          event "Disconnect": Value Change {
            # "UART Disconnect Button"
            n190 = event-data() -> ()  [unwired: 1 in, 3 out]
            n191 = Enqueue Element(queue=w544, element=CommandsV2.0."UART_Disconnect", error in (no error)=w543) -> (queue out=w546:refnum<queue>, error out=w545:errorcluster)  [unwired: 1 in, 1 out]
          }
        }
      }
    }
    frame #1 {
      n192 = Release Queue(queue=w547) -> ()  [unwired: 2 in, 3 out]
      n193 = Release Queue(queue=w549, error in (no error)=w548) -> ()  [unwired: 1 in, 3 out]
      n194 = Release Notifier(notifier=w550) -> ()  [unwired: 2 in, 3 out]
    }
  }
